vi "Set and Get ItemNames.vi"(7 "Mode":T1, 8 "错误输入":errorcluster, 10 "ItemNames In":string[](array[string]), 11 "Listbox Ref":refnum<vi>) -> (0 "错误输出":errorcluster, 2 "ItemNames Out":string[](array[string]), 3 "Dup Listbox Ref":refnum<vi>)   [LabVIEW 2012, in "Listbox Tool.lvlib"]
uses:
  Listbox Tool.lvlib
  Custom Type/Read and Write Mode.ctl
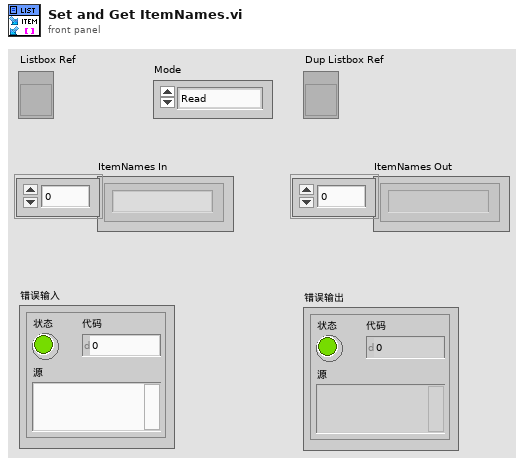
[diagram p1: front panel]
types:
  T1 = typedef "Listbox Tool.lvlib/Read and Write Mode.ctl" = enum16{"Read", "Write"}
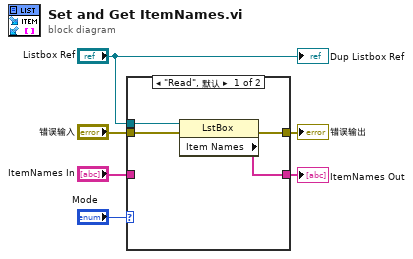
[diagram p0: block diagram]
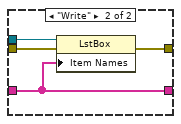
[diagram p2: hidden frame]
diagram:
  n1 = case shown="\"Read\", 默认" "Mode" {
    tunnel: "Listbox Ref" -> [w9 w14]
    tunnel: "错误输入" -> [w10 w13]
    tunnel: [w8 w12] -> w4
    tunnel: [w7 w11] -> w2
    tunnel: "ItemNames In" -> [_ w11]
    frame "Read", Default {
      n2 = property class="LstBox"(reference=w9, error in=w10) -> (error out=w8:errorcluster, "Item Names"=w7:string[])  [unwired: 1 out]
    }
    frame "Write" {
      n3 = property class="LstBox"(reference=w14, error in=w13, "Item Names"=w11) -> (error out=w12:errorcluster)  [unwired: 1 out]
    }
  }
  "错误输出" <- w4
  "ItemNames Out" <- w2
  "Dup Listbox Ref" <- "Listbox Ref"
